vi "Timeout.vi"(8 "error in (no error)":errorcluster, 11 "Turbo in":refnum<class "Turbo.lvclass">) -> (0 "error out":errorcluster, 3 "Turbo out":refnum<class "Turbo.lvclass">)   [LabVIEW 2015, in "cRIO-Carbondioxide.lvlib" / "CO2-Actor.lvlib" / "Turbo.lvclass"]
uses:
  Turbo.lvclass
  <instrlib>/BOC Edwards TIC/Turbo Instrument Controller.llb/Type Def - Pump State.ctl
  <instrlib>/BOC Edwards TIC/Turbo Instrument Controller.llb/Type Def - Alert ID.ctl
  <instrlib>/BOC Edwards TIC/Turbo Instrument Controller.llb/Type Def - Priority.ctl
  Turbo State Enumerator.ctl
  Turbo.lvclass/Turbo.ctl
  Valve Messages/Write Bit Field Msg/Write Bit Field Msg.lvclass/Write Bit Field Msg.ctl
  <vilib>/ActorFramework/Message Enqueuer/Message Enqueuer.lvclass/Message Enqueuer.ctl
  <vilib>/ActorFramework/Message Enqueuer/Enqueue.vi
  <vilib>/ActorFramework/Message Priority Queue/Priority Enqueue.vi
  CO2 Actor/CO2 Actor.lvclass
  Valve Messages/Write Bit Field Msg/Write Bit Field Msg.lvclass
  Interlocks/Interlock Chain/Interlock Chain.lvclass
panel:
  out "Turbo Pump State":T4 {"Gauge 1 Reading" format="%.2e"; "Pump Power (W)" format="%.1f"; "Pump Speed (%)" format="%.1f"}
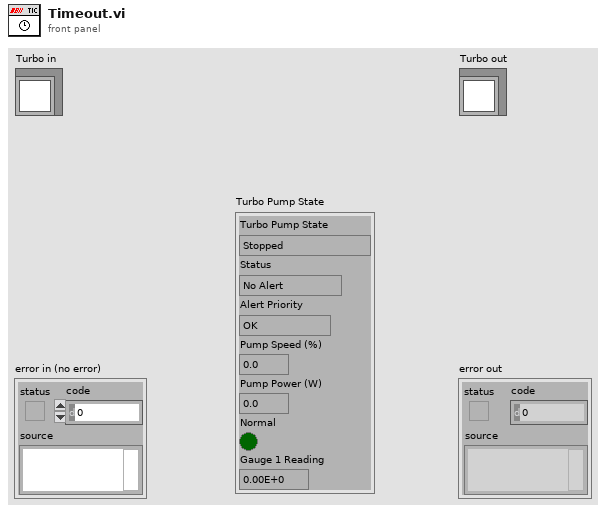
[diagram p1: front panel]
types:
  T1 = typedef "Type Def - Pump State.ctl" = enum16{"Stopped", "Starting Delay", "Stopping Short Delay", "Stopping Normal Delay", "Running", "Accelerating", "Fault Braking", "Braking"}
  T2 = typedef "Type Def - Alert ID.ctl" = enum16{"No Alert", "ADC Fault", "ADC Not Ready", "Over Range", "Under Range", "ADC Invalid", "No Gauge", "Unknown", "Not Supported", "New ID", "Ion EM Timeout", "Not Struck", "Filament Fail", "Mag Fail", "Striker Fail", "Cal Error", "Initialising", "Emission Error", "Over Pressure", "ASG Can't Zero", "Ramp Up Timeout", "Droop Timeout", "Run Hours High", "SC Interlock", "ID Volts Error", "Serial ID Fail", "Upload Active", "DX Fault", "Temp Alert", "SYSI Inhibit", "Ext Inhibit", "Temp Inhibit", "No Reading", "No Message", "NOV Failure", "ULoad Timeout", "DLoad Failed", "No Tube"}
  T3 = typedef "Type Def - Priority.ctl" = enum16{"OK", "Warning", "Alarm"}
  T4 = cluster{"Turbo Pump State":T1, "Status":T2, "Alert Priority":T3, "Pump Speed (%)":dbl, "Pump Power (W)":dbl, "Normal":bool, "Gauge 1 Reading":dbl}
  T5 = typedef "cRIO-Carbondioxide.lvlib/CO2-Actor.lvlib/Turbo.lvclass/Turbo State Enumerator.ctl" = enum16{"Undefined", "Error", "Abort", "Idle", "Initialize", "Start FV Pump", "Wait on FV Gauge", "Start Turbo", "Running", "Stop"}
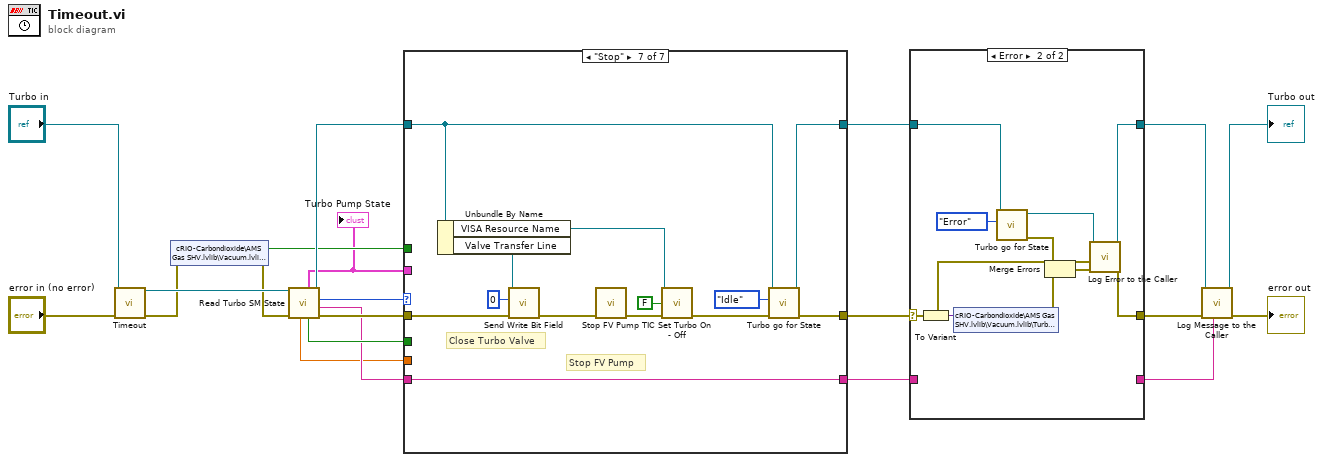
[diagram p0: block diagram]
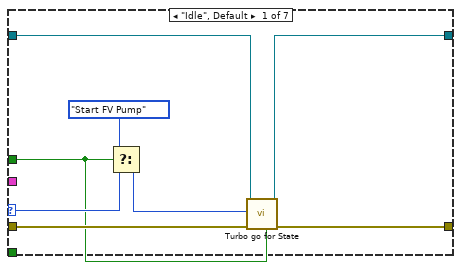
[diagram p3: hidden frame]
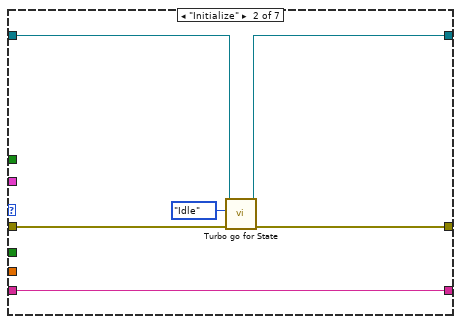
[diagram p4: hidden frame]
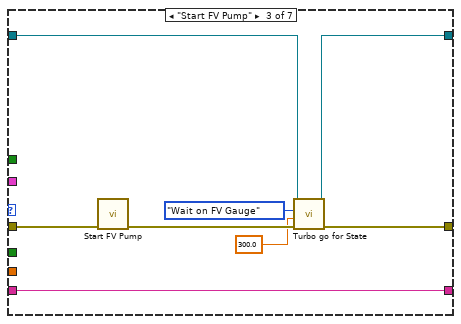
[diagram p5: hidden frame]
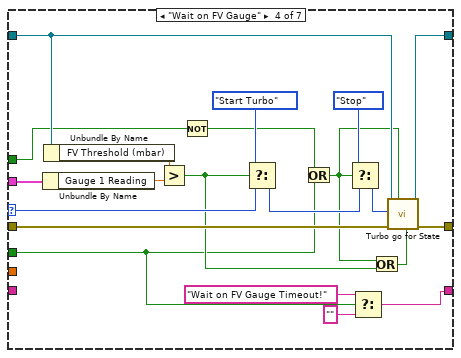
[diagram p6: hidden frame]
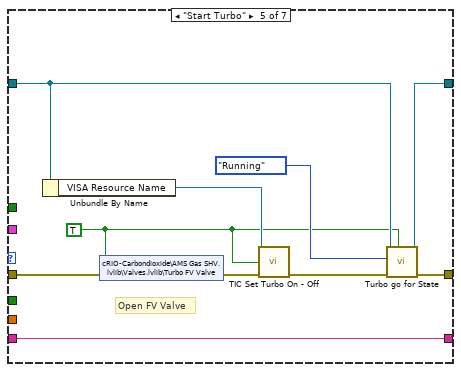
[diagram p7: hidden frame]
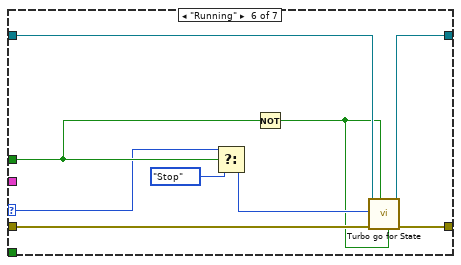
[diagram p8: hidden frame]
diagram:
  n1 = call-parent "Timeout.vi"("error in (no error)"="error in (no error)", "CO2 Actor in"="Turbo in") -> ("error out"=w12:errorcluster, "CO2 Actor out"=w19:refnum<class "Turbo.lvclass">)  [unwired: 8 in]
  n2 = shared-variable "cRIO-Carbondioxide\\AMS Gas SHV.lvlib\\Vacuum.lvlib\\Turbo ON"(error in=w12) -> (w10:bool, error out=w11:errorcluster)
  n3 = call "Read Turbo SM State.vi"("error in (no error)"=w11, "Turbo in"=w19) -> ("error out"=w18:errorcluster, "Sample Transfer State"=w14:string, "Turbo State"=w16:T5, "Turbo out"=w17:refnum<class "Turbo.lvclass">, "Timeout?"=w15:bool, "Turbo Pump State"=w8:T4, "State Timeout"=w7:dbl)  [unwired: 3 in]
  "Turbo Pump State" <- w8
  n4 = case shown="\"Stop\"" w16 {
    selector: w16 -> [w29 _ _ w55 _ w76 _]
    tunnel: w18 -> [w28 w35 w43 w61 w73 w83 w87]
    tunnel: [w27 w34 w41 w58 w70 w82 w93] -> w9
    tunnel: w17 -> [w26 w33 w40 w60 w69 w78 w89]
    tunnel: [w25 w32 w39 w59 w68 w77 w92] -> w13
    tunnel: w15 -> [_ _ _ w46 _ _ _]
    tunnel: w14 -> [_ w30 w36 _ w65 _ w90]
    tunnel: w10 -> [w22 _ _ w56 _ w79 _]
    tunnel: w8 -> [_ _ _ w64 _ _ _]
    tunnel: w7 -> [_ _ _ _ _ _ _]
    tunnel: [_ w30 w36 w47 w65 _ w90] -> w2
    frame "Idle", Default {
      n5 = Select(t=Turbo_State_Enumerator."Start FV Pump", s=w22, f=w29) -> (s? t:f=w24:T5)
      n6 = call "Turbo go for State.vi"("Publish? (T)"=w22, "error in (no error)"=w28, "Turbo State"=w24, "Turbo in"=w26) -> ("error out"=w27:errorcluster, "Turbo out"=w25:refnum<class "Turbo.lvclass">)  [unwired: 6 in]
    }
    frame "Initialize" {
      n7 = call "Turbo go for State.vi"("error in (no error)"=w35, "Turbo State"=Turbo_State_Enumerator."Idle", "Turbo in"=w33) -> ("error out"=w34:errorcluster, "Turbo out"=w32:refnum<class "Turbo.lvclass">)  [unwired: 7 in]
    }
    frame "Start FV Pump" {
      n8 = call "Start FV Pump.vi"("error in (no error)"=w43) -> ("error out"=w42:errorcluster)  [unwired: 10 in]
      n9 = call "Turbo go for State.vi"("error in (no error)"=w42, "State Timeout (Inf=no timeout )"=300.0, "Turbo State"=Turbo_State_Enumerator."Wait on FV Gauge", "Turbo in"=w40) -> ("error out"=w41:errorcluster, "Turbo out"=w39:refnum<class "Turbo.lvclass">)  [unwired: 6 in]
    }
    frame "Wait on FV Gauge" {
      n10 = Unbundle By Name(w64) -> ("Gauge 1 Reading"=w63:dbl)
      n11 = Unbundle By Name(w60) -> ("FV Threshold (mbar)"=w62:dbl)
      n12 = Greater?(x=w62, y=w63) -> (0:w53:bool)
      n13 = Not(x=w56) -> (.not. x?=w49:bool)
      n14 = Select(t=Turbo_State_Enumerator."Start Turbo" ("Turbo State"), s=w53, f=w55) -> (s? t:f=w51:T5)
      n15 = Or(x=w49, y=w46) -> (x .or. y?=w48:bool)
      n16 = Select(t=Turbo_State_Enumerator."Stop" ("f"), s=w48, f=w51) -> (s? t:f=w50:T5)
      n17 = Select(t="Wait on FV Gauge Timeout!", s=w46, f="") -> (s? t:f=w47:string)
      n18 = Or(x=w48, y=w53) -> (x .or. y?=w57:bool)
      n19 = call "Turbo go for State.vi"("Publish? (T)"=w57, "Immediately (false = stick to schedule)"=w48, "error in (no error)"=w61, "Turbo State"=w50, "Turbo in"=w60) -> ("error out"=w58:errorcluster, "Turbo out"=w59:refnum<class "Turbo.lvclass">)  [unwired: 5 in]
    }
    frame "Start Turbo" {
      w66 = TRUE ("Turbo FV valve")
      # "Open FV Valve"
      n20 = Unbundle By Name(w69) -> ("VISA Resource Name"=w72:refnum<visa-resource-name>)
      n21 = shared-variable "cRIO-Carbondioxide\\AMS Gas SHV.lvlib\\Valves.lvlib\\Turbo FV Valve"(w66, error in=w73) -> (error out=w74:errorcluster)
      n22 = call <instrlib>:"TIC Set Turbo On - Off.vi"("VISA Session In"=w72, "On (F)"=w66, "error in (no error)"=w74) -> ("error out"=w71:errorcluster)  [unwired: 11 in, 1 out]
      n23 = call "Turbo go for State.vi"("Immediately (false = stick to schedule)"=w66, "error in (no error)"=w71, "Turbo State"=Turbo_State_Enumerator."Running", "Turbo in"=w69) -> ("error out"=w70:errorcluster, "Turbo out"=w68:refnum<class "Turbo.lvclass">)  [unwired: 6 in]
    }
    frame "Running" {
      n24 = Select(t=w76, s=w79, f=Turbo_State_Enumerator."Stop") -> (s? t:f=w81:T5)
      n25 = Not(x=w79) -> (.not. x?=w75:bool)
      n26 = call "Turbo go for State.vi"("Publish? (T)"=w75, "Immediately (false = stick to schedule)"=w75, "error in (no error)"=w83, "Turbo State"=w81, "Turbo in"=w78) -> ("error out"=w82:errorcluster, "Turbo out"=w77:refnum<class "Turbo.lvclass">)  [unwired: 5 in]
    }
    frame "Stop" {
      # "Close Turbo Valve"
      # "Stop FV Pump"
      n27 = Unbundle By Name(w89) -> ("VISA Resource Name"=w88:refnum<visa-resource-name>, "Valve Transfer Line"=w85:refnum<class "Message Enqueuer.lvclass">)
      n28 = call "Send Write Bit Field.vi"("error in (no error)"=w87, "Bit Field"=u16 0, "Message Enqueuer"=w85) -> ("error out"=w86:errorcluster)  [unwired: 5 in, 3 out]
      n29 = call "Stop FV Pump.vi"("error in (no error)"=w86) -> ("error out"=w96:errorcluster)  [unwired: 10 in]
      n30 = call <instrlib>:"TIC Set Turbo On - Off.vi"("VISA Session In"=w88, "On (F)"=FALSE, "error in (no error)"=w96) -> ("error out"=w94:errorcluster)  [unwired: 11 in, 1 out]
      n31 = call "Turbo go for State.vi"("error in (no error)"=w94, "Turbo State"=Turbo_State_Enumerator."Idle", "Turbo in"=w89) -> ("error out"=w93:errorcluster, "Turbo out"=w92:refnum<class "Turbo.lvclass">)  [unwired: 7 in]
    }
  }
  n32 = case shown="Error" w9 {
    selector: w9 -> [w99 w102]
    tunnel: [w99 w100] -> w6
    tunnel: w13 -> [w98 w108]
    tunnel: [w98 w104] -> w4
    tunnel: [w97 _] -> w1
    tunnel: w2 -> [w97 _]
    frame No Error {
    }
    frame Error {
      n33 = To Variant(anything=w102) -> (Variant=w109:variant)
      n34 = shared-variable "cRIO-Carbondioxide\\AMS Gas SHV.lvlib\\Vacuum.lvlib\\Turbo Error"(w109) -> (error out=w105:errorcluster)  [unwired: 1 in]
      n35 = call "Turbo go for State.vi"("Turbo State"=Turbo_State_Enumerator."Error", "Turbo in"=w108) -> ("error out"=w106:errorcluster, "Turbo out"=w103:refnum<class "Turbo.lvclass">)  [unwired: 8 in]
      n36 = Merge Errors(w106, w105) -> (w101:errorcluster)
      n37 = call-dynamic "Log Error to the Caller.vi"("error in (no error)"=w101, "Error to log"=w102, "CO2 Actor in"=w103) -> ("error out"=w100:errorcluster, "CO2 Actor out"=w104:refnum<class "Turbo.lvclass">)  [unwired: 7 in]
    }
  }
  n38 = call-dynamic "Log Message to the Caller.vi"("String (\"\" = no message to send)"=w1, "error in (no error)"=w6, "CO2 Actor in"=w4) -> ("error out"=→"error out":errorcluster, "CO2 Actor out"=→"Turbo out":refnum<class "Turbo.lvclass">)  [unwired: 7 in]
